vi "HOR_SCALE_SETTING.vi"(0 "VISA TDS1012":refnum<visa-resource-name>="GPIB0::1::INSTR", 1 "HOR_SCAIL":string) -> ()   [LabVIEW 2018]
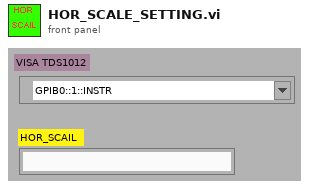
[diagram p1: front panel]
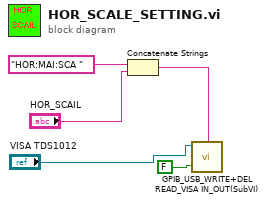
[diagram p0: block diagram]
diagram:
  n1 = Concatenate Strings("HOR:MAI:SCA ", "HOR_SCAIL") -> (w2:string)
  n2 = call "GPIB_USB_WRITE+DEL READ_VISA IN_OUT(SubVI).vi"("VISA resource IN"="VISA TDS1012", "GPIB/USB WRITE"=w2, 4:FALSE ("READ GPIB")) -> ()  [unwired: 3 in, 3 out]
